vi "get_callbackVisitors.vi"(0 "HGF_NetworkEvent":refnum<class "HGF_NetworkEvent.lvclass">, 5 "error in (no error)":errorcluster) -> (14 "dup HGF_NetworkEvent":refnum<class "HGF_NetworkEvent.lvclass">, 16 "callbackVisitors":refnum<class "HGF_NetworkVisitor.lvclass">[](array[class]), 19 "error out":errorcluster)   [LabVIEW 2014, in "HGF_BaseClasses.lvlib" / "HGF_NetworkEvent.lvclass"]
doc: "This VI returns the network callback Visitors."
uses:
  HGF_NetworkEvent.lvclass
  HGF_NetworkVisitor/HGF_NetworkVisitor.lvclass
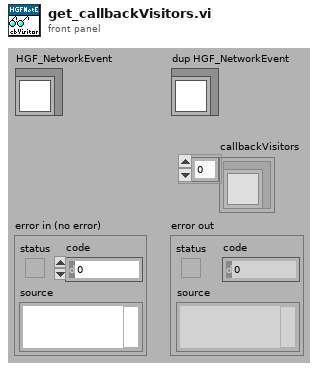
[diagram p1: front panel]
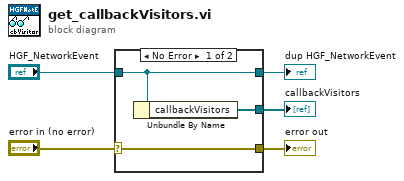
[diagram p0: block diagram]
diagram:
  n1 = case shown="No Error" "error in (no error)" {
    selector: "error in (no error)" -> [w8 w9]
    tunnel: [w8 w9] -> w4
    tunnel: [w7 w10] -> w2
    tunnel: "HGF_NetworkEvent" -> [w7 w10]
    tunnel: [w6 _] -> w1
    frame No Error {
      n2 = Unbundle By Name(w7) -> ("callbackVisitors"=w6:refnum<class "HGF_NetworkVisitor.lvclass">[])
    }
    frame Error {
    }
  }
  "error out" <- w4
  "dup HGF_NetworkEvent" <- w2
  "callbackVisitors" <- w1
